vi "ecg(SubVI).vi"(11 "nb de période":dbl) -> (3 "signal out":waveform(dbl))   [LabVIEW 2018]
uses:
  <vilib>/measure/NI_MABase.lvlib
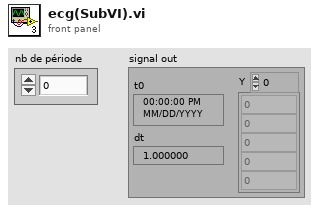
[diagram p1: front panel]
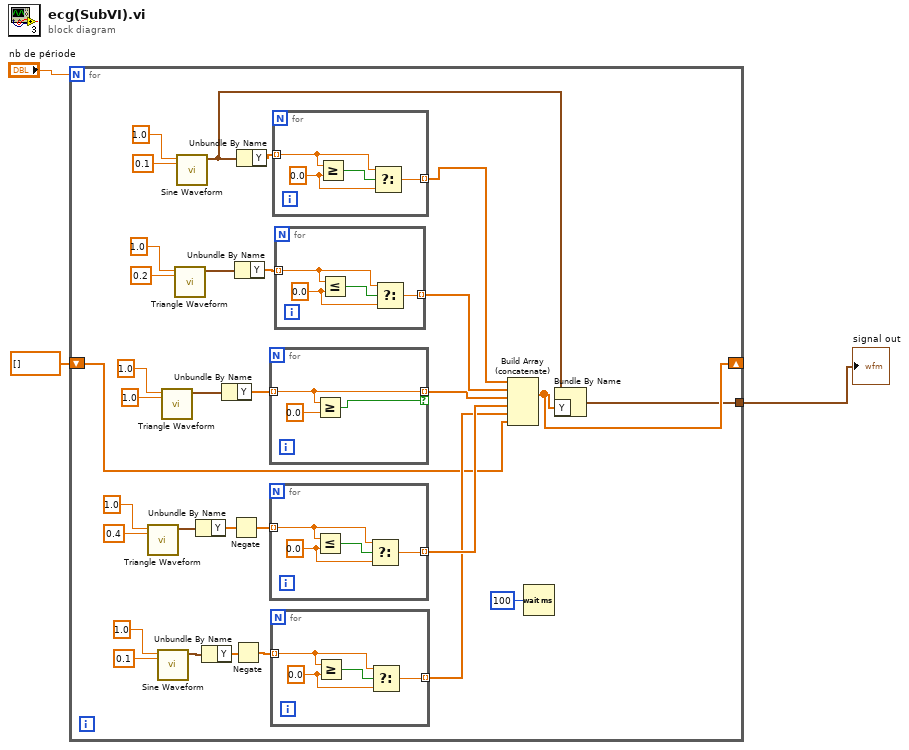
[diagram p0: block diagram]
diagram:
  n1 = for {
    N: "nb de période" -> [_]
    shift-right: [w6] -> _
    shift-left: dbl[] [] -> [w7]
    tunnel: [w4] -> w2
    n2 = call <vilib>:"Triangle Waveform.vi"("amplitude"=0.4, "frequency"=1.0) -> ("signal out"=w25:waveform(dbl))  [unwired: 8 in, 1 out]
    n3 = call <vilib>:"Sine Waveform.vi"("amplitude"=0.1, "frequency"=1.0) -> ("signal out"=w17:waveform(dbl))  [unwired: 8 in, 1 out]
    n4 = call <vilib>:"Triangle Waveform.vi"("amplitude"=1.0, "frequency"=1.0) -> ("signal out"=w21:waveform(dbl))  [unwired: 8 in, 1 out]
    n5 = call <vilib>:"Triangle Waveform.vi"("amplitude"=0.2, "frequency"=1.0) -> ("signal out"=w10:waveform(dbl))  [unwired: 8 in, 1 out]
    n6 = call <vilib>:"Sine Waveform.vi"("amplitude"=0.1, "frequency"=1.0) -> ("signal out"=w9:waveform(dbl))  [unwired: 8 in, 1 out]
    n7 = Unbundle By Name(w25) -> ("Y"=w26:dbl[])
    n8 = Unbundle By Name(w17) -> ("Y"=w18:dbl[])
    n9 = Unbundle By Name(w21) -> ("Y"=w22:dbl[])
    n10 = Negate(x=w26) -> (-x=w8:dbl[])
    n11 = Negate(x=w18) -> (-x=w16:dbl[])
    n12 = Unbundle By Name(w10) -> ("Y"=w29:dbl[])
    n13 = Unbundle By Name(w9) -> ("Y"=w32:dbl[])
    n14 = for {
      tunnel: w22 -> [w40] mode=indexing
      tunnel: [w40] -> w13 mode=indexing if=w39
      n15 = Greater Or Equal?(x=w40, y=0.0) -> (x >= y?=w39:bool)
    }
    n16 = for {
      tunnel: w8 -> [w45] mode=indexing
      tunnel: [w42] -> w12 mode=indexing
      w44 = 0.0 ("y")
      n17 = Less Or Equal?(x=w45, y=w44) -> (x <= y?=w43:bool)
      n18 = Select(t=w45, s=w43, f=w44) -> (s? t:f=w42:dbl)
    }
    n19 = for {
      tunnel: w16 -> [w38] mode=indexing
      tunnel: [w35] -> w11 mode=indexing
      w37 = 0.0 ("y")
      n20 = Greater Or Equal?(x=w38, y=w37) -> (x >= y?=w36:bool)
      n21 = Select(t=w38, s=w36, f=w37) -> (s? t:f=w35:dbl)
    }
    n22 = for {
      tunnel: w32 -> [w53] mode=indexing
      tunnel: [w50] -> w15 mode=indexing
      w52 = 0.0 ("y")
      n23 = Greater Or Equal?(x=w53, y=w52) -> (x >= y?=w51:bool)
      n24 = Select(t=w53, s=w51, f=w52) -> (s? t:f=w50:dbl)
    }
    n25 = for {
      tunnel: w29 -> [w49] mode=indexing
      tunnel: [w46] -> w14 mode=indexing
      w48 = 0.0 ("y")
      n26 = Less Or Equal?(x=w49, y=w48) -> (x <= y?=w47:bool)
      n27 = Select(t=w49, s=w47, f=w48) -> (s? t:f=w46:dbl)
    }
    n28 = Build Array (concatenate)(w15, w14, w13, w12, w11, w7) -> (w6:dbl[])
    n29 = Wait (ms)(milliseconds to wait=u32 100) -> ()  [unwired: 1 out]
    n30 = Bundle By Name(cluster=w9, "Y"=w6) -> (w4:waveform(dbl))
  }
  "signal out" <- w2
